vi "Practica3.4_Case.vi"() -> ()   [LabVIEW 2022 SP3]
panel:
  in  "Selector numérico":dbl
  out "Valor numérico":dbl(knob) scale=0.0..10.0
  out "?":bool
  out "?":bool
  out "?":bool
  out "?":bool
  out "?":bool
  out "?":bool
  out "?":bool
  # "Anahí Montserrat Vázquez Padilla \nPráctica 03: Case \n31/01/2024"
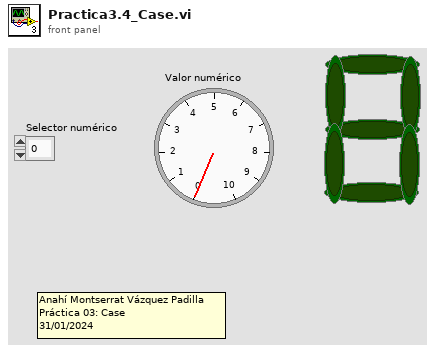
[diagram p1: front panel]
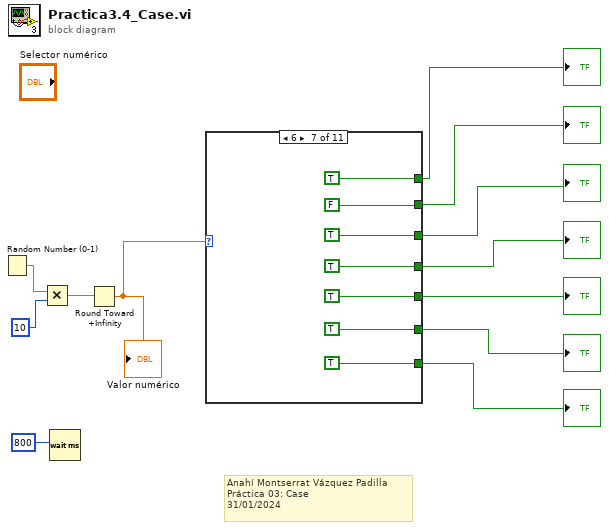
[diagram p0: block diagram]
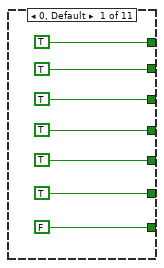
[diagram p2: hidden frame]
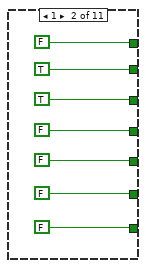
[diagram p3: hidden frame]
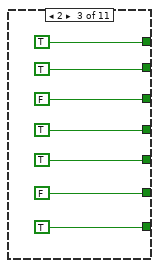
[diagram p4: hidden frame]
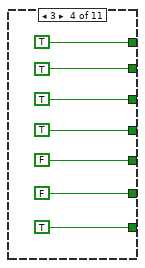
[diagram p5: hidden frame]
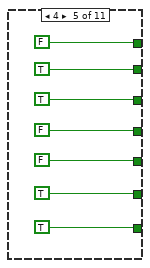
[diagram p6: hidden frame]
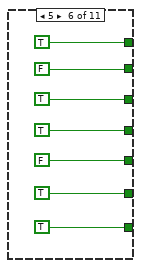
[diagram p7: hidden frame]
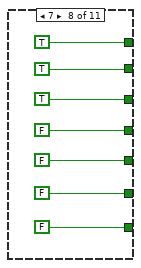
[diagram p8: hidden frame]
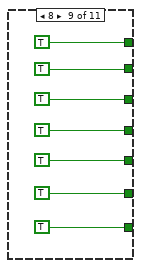
[diagram p9: hidden frame]
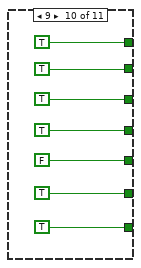
[diagram p10: hidden frame]
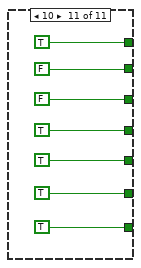
[diagram p11: hidden frame]
diagram:
  # "Anahí Montserrat Vázquez Padilla \nPráctica 03: Case \n31/01/2024"
  n1 = Random Number (0-1)() -> (number: 0 to 1=w5:dbl)
  n2 = Multiply(x=w5, y=10) -> (x*y=w3:dbl)
  n3 = Wait (ms)(milliseconds to wait=800) -> ()  [unwired: 1 out]
  n4 = Round Toward +Infinity(x=w3) -> (ceil(x): smallest int >= x=w2:dbl)
  "Valor numérico" <- w2
  n5 = case shown="6" w2 {
    tunnel: [TRUE FALSE TRUE TRUE FALSE TRUE TRUE TRUE TRUE TRUE TRUE] -> w12
    tunnel: [TRUE TRUE TRUE TRUE TRUE FALSE FALSE TRUE TRUE TRUE FALSE] -> w11
    tunnel: [TRUE TRUE FALSE TRUE TRUE TRUE TRUE TRUE TRUE TRUE FALSE] -> w10
    tunnel: [TRUE FALSE TRUE TRUE FALSE TRUE TRUE FALSE TRUE TRUE TRUE] -> w9
    tunnel: [TRUE FALSE TRUE FALSE FALSE FALSE TRUE FALSE TRUE FALSE TRUE] -> w8
    tunnel: [TRUE FALSE FALSE FALSE TRUE TRUE TRUE FALSE TRUE TRUE TRUE] -> w7
    tunnel: [FALSE FALSE TRUE TRUE TRUE TRUE TRUE FALSE TRUE TRUE TRUE] -> w6
    frame 0, Default {
    }
    frame 1 {
    }
    frame 2 {
    }
    frame 3 {
    }
    frame 4 {
    }
    frame 5 {
    }
    frame 6 {
    }
    frame 7 {
    }
    frame 8 {
    }
    frame 9 {
    }
    frame 10 {
    }
  }
  "?" <- w12
  "?" <- w6
  "?" <- w9
  "?" <- w11
  "?" <- w10
  "?" <- w7
  "?" <- w8
